vi "Evaluate.vi"(0 "BallInterception in":refnum<class "ShotInterception.lvclass">, 2 "Point":dbl[](array[numeric]), 3 "Ally?":bool, 4 "GameRef":refnum<data-value>, 5 "error in (no error)":errorcluster) -> (14 "BallInterception out":refnum<class "ShotInterception.lvclass">, 16 "Evaluation":dbl, 19 "error out":errorcluster)   [LabVIEW 2023, in "ShotInterception.lvclass"]
uses:
  ShotInterception.lvclass
  Game_class/Game.lvclass
  Game_class/Game.lvclass/Game.ctl
  Referee_class/Referee.lvclass/Referee.ctl
  Team_class/Team.lvclass/Team.ctl
  Field_class/Field.lvclass/Field.ctl
  Robot_class/Robot.lvclass/Robot.ctl
  Object_class/Object.lvclass/Object.ctl
  <vilib>/Analysis/coordinate.llb/2D Cartesian Coordinate Shift (Scalar).vi
  <vilib>/Analysis/coordinate.llb/2D Cartesian Coordinate Rotation (Scalar).vi
  Robot_class/Read id.vi
  Object_class/Read position(x,y).vi
  Game_class/Read Referee.vi
  Game_class/Read EnemyRef.vi
  Game_class/Read BallRef.vi
  Game_class/Read Utilities.lvclass.vi
  Game_class/Read FieldRef.vi
  Field_class/Read enemyGoalPosition.vi
  Field_class/Read ourGoalPosition.vi
  Team_class/Read RobotRef.vi
  Referee_class/Read enemy_goalie_id.vi
  Enemy_class/Enemy.lvclass
  C:/Users/ebert/Documents/codes/SSL/repo/SSL_AI/Team_class/Team.lvclass
  Robot_class/Robot.lvclass
  C:/Users/ebert/Documents/codes/SSL/repo/SSL_AI/Object_class/Object.lvclass
  Referee_class/Referee.lvclass
  Ball_class/Ball.lvclass
  Utilities_class/Utilities.lvclass
  Field_class/Field.lvclass
  <vilib>/Analysis/NI_AALPro.lvlib
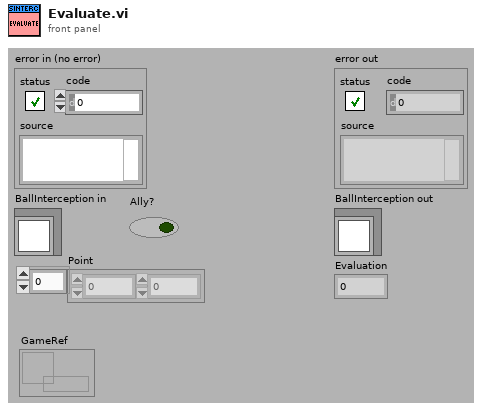
[diagram p1: front panel]
types:
  T1 = typedef "STPParameters.ctl" = cluster{"Skills":T2, "TestSkill":T4, "Events":cluster{"distanceToBallPossession":dbl, "timeForPossessionThreshold":dbl}, "Criteria":cluster{"OpenAngleToGoal":cluster{"minAngle":dbl, "maxAngle":dbl, "minEvaluation":dbl}, "PassDistance":cluster{"maxDistance":dbl, "minDistance":dbl}, "ShotInterception":cluster{"shotSpeed":dbl, "minEnemySpeed":dbl, "minEvaluation":dbl, "maxEnemySpeed":dbl}, "OneTouchShot":cluster{"MaxAngle":dbl, "minEvaluation":dbl}, "PassInterception":cluster{"minEnemySpeed":dbl, "maxEnemySpeed":dbl, "chipPassDistance":dbl, "chipPassEval":dbl, "minEvaluation":dbl}}, "minPassSpeed":dbl, "maxPassSpeed":dbl, "AllyTeamIds":T5[], "ReceiverSpeed":dbl, "minEvaluationToShoot":dbl}
  T2 = typedef "Skills.ctl" = cluster{"CirculateBall":T3, "ProtectBall":cluster{"DistanceFromBall":dbl}}
  T3 = typedef "CIrculateSkillParameters.ctl" = cluster{"rotationAngle":dbl, "velocityFactor":dbl, "OrientationFactor":dbl}
  T4 = typedef "TestSkills.ctl" = enum16{"AlignSkill", "PassSkill", "CirculateBall", "OneTouchShotSkill", "KickToSkill_v2", "ShootSkill", "InterceptBall", "Exit", "GoToSkill_v2"}
  T5 = typedef "AllyTeam.ctl" = enum16{"Keeper", "Defender", "Attacker"}
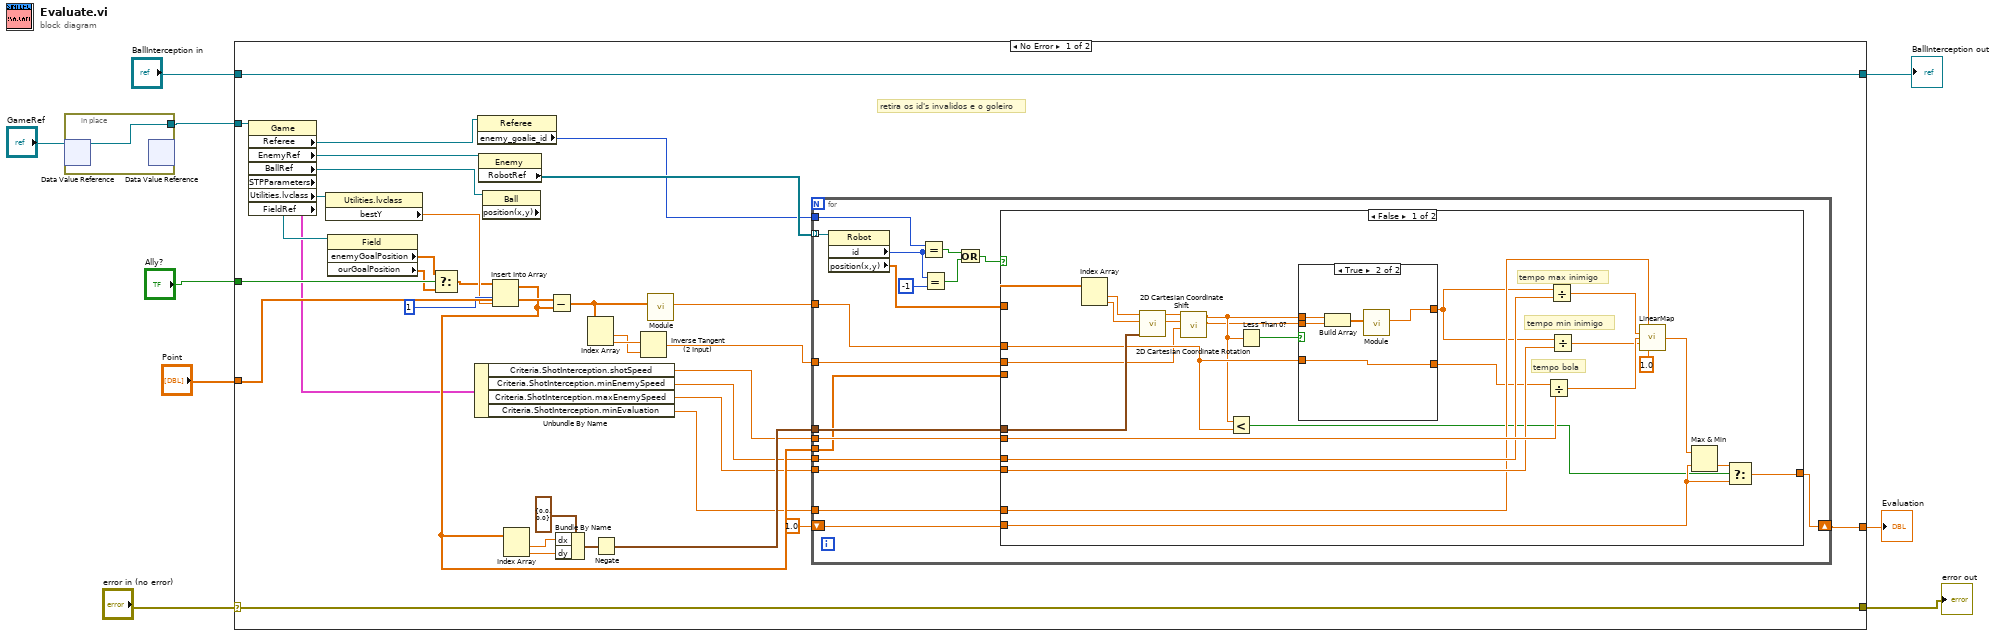
[diagram p0: block diagram]
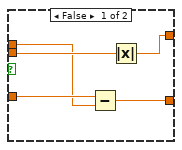
[diagram p2: hidden frame]
diagram:
  n1 = in-place {
    in-place-border: [w10] -> w2
    n2 = in-place-dvr #1("GameRef") -> (w10:refnum<class "Game.lvclass">)  [unwired: 1 out]
    n3 = in-place-dvr #1() -> ()  [unwired: 1 in, 2 out]
  }
  n4 = case shown="No Error" "error in (no error)" {
    selector: "error in (no error)" -> [w45 w102]
    tunnel: [w45 w102] -> w4
    tunnel: "BallInterception in" -> [w44 w101]
    tunnel: [w44 w101] -> w6
    tunnel: w2 -> [w43 _]
    tunnel: "Point" -> [w24 _]
    tunnel: [w28 _] -> w8
    tunnel: "Ally?" -> [w19 _]
    frame No Error {
      # "retira os id's invalidos e o goleiro"
      n5 = property class="Game"(reference=w43) -> ("Referee"=w40:refnum<class "Referee.lvclass">, "EnemyRef"=w42:refnum<class "Enemy.lvclass">, "BallRef"=w38:refnum<class "Ball.lvclass">, "STPParameters"=w15:T1, "Utilities.lvclass"=w25:refnum<class "Utilities.lvclass">, "FieldRef"=w23:refnum<class "Field.lvclass">)  [unwired: 1 in, 2 out]
      n6 = property class="Utilities.lvclass"(reference=w25) -> ("bestY"=w21:dbl)  [unwired: 1 in, 2 out]
      n7 = property class="Field"(reference=w23) -> ("enemyGoalPosition"=w17:dbl[], "ourGoalPosition"=w16:dbl[])  [unwired: 1 in, 2 out]
      n8 = Select(t=w17, s=w19, f=w16) -> (s? t:f=w18:dbl[])
      n9 = Unbundle By Name(w15) -> ("Criteria.ShotInterception.shotSpeed"=w14:dbl, "Criteria.ShotInterception.minEnemySpeed"=w13:dbl, "Criteria.ShotInterception.maxEnemySpeed"=w12:dbl, "Criteria.ShotInterception.minEvaluation"=w11:dbl)
      n10 = property class="Referee"(reference=w40) -> ("enemy_goalie_id"=w39:i32)  [unwired: 1 in, 2 out]
      n11 = property class="Enemy"(reference=w42) -> ("RobotRef"=w41:refnum<class "Robot.lvclass">[])  [unwired: 1 in, 2 out]
      n12 = property class="Ball" props=["position(x,y)"](reference=w38) -> ()  [unwired: 1 in, 3 out]
      n13 = Insert Into Array(array=w18, index=1, new element=w21) -> (w20:dbl[])
      n14 = Index Array(array=w20) -> (element #1=w33:dbl, element #2=w32:dbl)  [unwired: 2 in]
      n15 = Subtract(x=w24, y=w20) -> (x-y=w31:dbl[])
      n16 = Bundle By Name(cluster=cluster{"dx":dbl, "dy":dbl} {"dx"=0.0, "dy"=0.0} ("shift"), "dx"=w33, "dy"=w32) -> (w27:cluster{"dx":dbl, "dy":dbl})
      n17 = Index Array(array=w31) -> (element #1=w36:dbl, element #2=w37:dbl)  [unwired: 2 in]
      n18 = Negate(x=w27) -> (-x=w26:cluster{"dx":dbl, "dy":dbl})
      n19 = Inverse Tangent (2 Input)(1:w36, 2:w37) -> (0:w35:dbl)
      n20 = call "Module.vi"("2D vector"=w31) -> ("Modulo"=w30:dbl)  [unwired: 8 in, 2 out]
      n21 = for {
        tunnel: w41 -> [w63] mode=indexing
        tunnel: w39 -> [w49]
        tunnel: w35 -> [w62]
        tunnel: w26 -> [w60]
        tunnel: w30 -> [w59]
        tunnel: w14 -> [w58]
        shift-right: [w56] -> w28
        shift-left: 1.0 ("Numeric") -> [w57]
        tunnel: w20 -> [w55]
        tunnel: w13 -> [w54]
        tunnel: w12 -> [w53]
        tunnel: w11 -> [w52]
        n22 = property class="Robot"(reference=w63) -> ("id"=w50:i32, "position(x,y)"=w61:dbl[])  [unwired: 1 in, 2 out]
        n23 = Equal?(x=w49, y=w50) -> (x = y?=w48:bool)
        n24 = Equal?(x=w50, y=-1 ("x")) -> (x = y?=w47:bool)
        n25 = Or(x=w48, y=w47) -> (x .or. y?=w46:bool)
        n26 = case shown="False" w46 {
          tunnel: w62 -> [w81 _]
          tunnel: w61 -> [w87 _]
          tunnel: w60 -> [w89 _]
          tunnel: w59 -> [w85 _]
          tunnel: w58 -> [w86 _]
          tunnel: w57 -> [w82 w100]
          tunnel: [w88 w100] -> w56
          tunnel: w55 -> [_ _]
          tunnel: w54 -> [w84 _]
          tunnel: w53 -> [w83 _]
          tunnel: w52 -> [w80 _]
          frame False {
            # "tempo bola"
            # "tempo min inimigo"
            # "tempo max inimigo"
            n27 = Index Array(array=w87) -> (element #1=w69:dbl, element #2=w68:dbl)  [unwired: 2 in]
            n28 = call-poly <vilib>:"2D Cartesian Coordinate Shift.vi"("shift"=w89, "y"=w68, "x"=w69) -> ("y out"=w66:dbl, "x out"=w67:dbl)  [unwired: 6 in, 1 out]
            n29 = call-poly <vilib>:"2D Cartesian Coordinate Rotation.vi"("theta"=w81, "y"=w66, "x"=w67) -> ("y out"=w64:dbl, "x out"=w65:dbl)  [unwired: 6 in, 1 out]
            n30 = Less?(x=w65, y=w85) -> (x < y?=w78:bool)
            n31 = Less Than 0?(x=w65) -> (x < 0?=w79:bool)
            n32 = case shown="True" w79 {
              tunnel: w65 -> [w90 w97]
              tunnel: w64 -> [w93 w95]
              tunnel: [w92 w99] -> w75
              tunnel: w85 -> [w91 w98]
              tunnel: [w94 w98] -> w74
              frame False {
                n33 = Subtract(x=w91, y=w90) -> (x-y=w94:dbl)
                n34 = Absolute Value(x=w93) -> (abs(x)=w92:dbl)
              }
              frame True {
                n35 = Build Array(w97, w95) -> (w96:dbl[])
                n36 = call "Module.vi"("2D vector"=w96) -> ("Modulo"=w99:dbl)  [unwired: 8 in, 2 out]
              }
            }
            n37 = Divide(x=w74, y=w86) -> (x/y=w77:dbl)
            n38 = Divide(x=w75, y=w84) -> (x/y=w73:dbl)
            n39 = Divide(x=w75, y=w83) -> (x/y=w72:dbl)
            n40 = call "LinearMap.vi"("MaxY"=w80, "MaxX"=w73, "X"=w77, "MinX"=w72, "MinY"=1.0) -> ("Y"=w71:dbl)  [unwired: 8 in, 2 out]
            n41 = Max & Min(x=w71, y=w82) -> (min(x,y)=w70:dbl)  [unwired: 1 out]
            n42 = Select(t=w70, s=w78, f=w82) -> (s? t:f=w88:dbl)
          }
          frame True {
          }
        }
      }
    }
    frame Error {
    }
  }
  "error out" <- w4
  "BallInterception out" <- w6
  "Evaluation" <- w8
